vi "form_live_viewer_2D.vi"(11 "JSON":string="{\"ch\":0}") -> ()   [LabVIEW 2021]
uses:
  <vilib>/Analysis/baseanly.llb/Mean (DBL).vi
  core/host_global_vars.vi
  <vilib>/Analysis/NI_AALBase.lvlib
panel:
  in  "Line offset":bool
  in  "Ring":u16(ring) items=["AI 0", "AI 1", "AI 2", "AI 3", "AI 4", "AI 5", "AI 6", "AI 7", "AO 0", "AO 1", "AO 2", "AO 3", "AO 4", "AO 5", "AO 6", "AO 7", "FB 0", "FB 1", "FB 0 error", "FB 1 error"]
  in  "fargs":cluster{"ch":i32}
  out "Intensity Graph":dbl[][](graph)
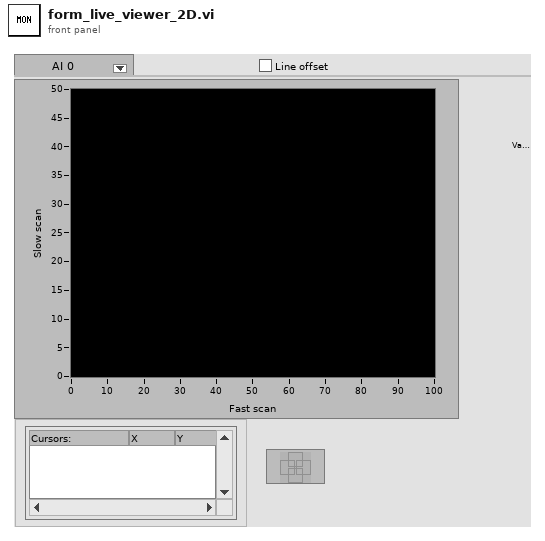
[diagram p1: front panel]
types:
  T1 = typedef "fpga_dtype_index.ctl" = cluster{"page":i16, "2nd":i16, "1st":i16}
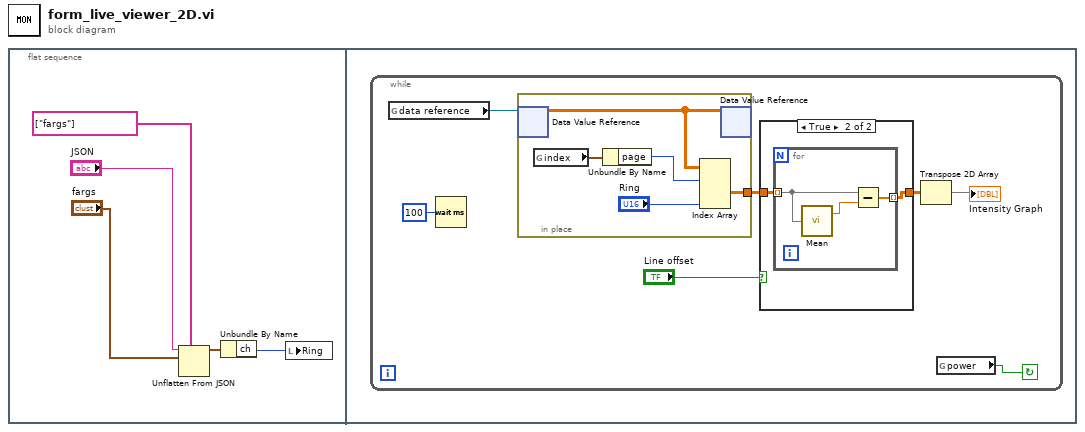
[diagram p0: block diagram]
diagram:
  n1 = flat-sequence {
    frame #0 {
      n2 = Unflatten From JSON(path=string[] ["fargs"], JSON string="JSON", type and defaults="fargs") -> (value=w4:cluster{"ch":i32})  [unwired: 4 in, 1 out]
      n3 = Unbundle By Name(w4) -> ("ch"=w5:i32)
      n4 = local write "Ring"(w5) -> ()
    }
    frame #1 {
      n5 = while {
        stop <- w11 continue-if-true
        n6 = global read "host_global_vars.vi" "data reference"() -> (w12:refnum<data-value>)
        n7 = Wait (ms)(milliseconds to wait=u32 100) -> ()  [unwired: 1 out]
        n8 = in-place {
          in-place-border: [w21] -> w9
          n9 = in-place-dvr #1(w12) -> (w23:sgl[][][][])  [unwired: 1 out]
          n10 = global read "host_global_vars.vi" "index"() -> (w20:T1)
          n11 = Unbundle By Name(w20) -> ("page"=w19:i16)
          n12 = Index Array(array=w23, index (dim 0)=w19, index (dim 3)="Ring") -> (element=w21:sgl[][])  [unwired: 2 in]
          n13 = in-place-dvr #1(w23) -> ()  [unwired: 2 out]
        }
        n14 = case shown="True" "Line offset" {
          tunnel: w9 -> [w13 w15]
          tunnel: [w13 w14] -> w7
          frame False {
          }
          frame True {
            n15 = for {
              tunnel: w15 -> [w17] mode=indexing
              tunnel: [w16] -> w14 mode=indexing
              n16 = call-poly <vilib>:"Mean.vi"("X"=w17) -> ("mean"=w18:dbl)  [unwired: 1 out]
              n17 = Subtract(x=w17, y=w18) -> (x-y=w16:dbl[])
            }
          }
        }
        n18 = Transpose 2D Array(2D array=w7) -> (transposed array=→"Intensity Graph":dbl[][])
        n19 = global read "host_global_vars.vi" "power"() -> (w11:bool)
      }
    }
  }
